vi "Kerosene_Pressure.vi"() -> ()   [LabVIEW 2018]
panel:
  in  "End Loop":bool
  out "?":dbl
  out "Kerosene Pressure":dbl(knob) scale=0.0..1500.0
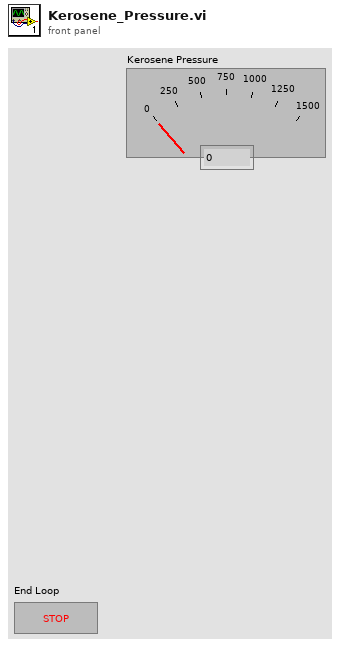
[diagram p1: front panel]
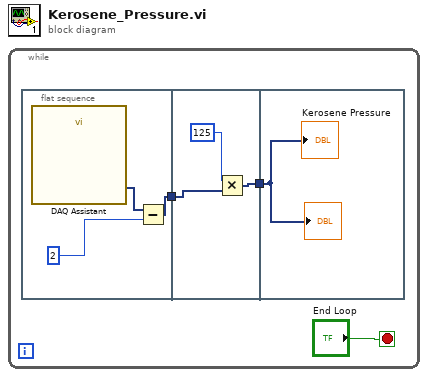
[diagram p0: block diagram]
diagram:
  n1 = while {
    stop <- "End Loop" stop-if-true
    n2 = flat-sequence {
      tunnel: [w5] -> w3
      tunnel: w3 -> [w9]
      tunnel: [w7] -> w2
      tunnel: w2 -> [w10]
      frame #0 {
        n3 = call "DAQ Assistant"() -> ("data"=w4:dynamicdata)  [unwired: 17 in, 2 out]
        n4 = Subtract(x=w4, y=2) -> (x-y=w5:dynamicdata)
      }
      frame #1 {
        n5 = Multiply(x=125, y=w9) -> (x*y=w7:dynamicdata)
      }
      frame #2 {
        "Kerosene Pressure" <- w10
        "?" <- w10
      }
    }
  }
